vi "Test Configure.vi"(0 "niDTS BT Rx Test in":refnum<class "niDTS BT Rx Test.lvclass">, 11 "error in (no error)":errorcluster) -> (4 "niDTS BT Rx Test out":refnum<class "niDTS BT Rx Test.lvclass">, 15 "error out":errorcluster)   [LabVIEW 2015, in "niDTS BT.lvlib" / "niDTS BT Rx Test.lvclass"]
uses:
  niDTS BT Rx Test.lvclass
  Includes/niDTS BT DUT INC Parameters.ctl
  RiviInstDriver/niRfsgBT/Includes/niRfsgBt INC Handle.ctl
  RiviInstDriver/niRfsgBT/Objects/niRfsgBt.lvclass
  niDTS BT Rx Test.lvclass/niDTS BT Rx Test.ctl
  RiviInstDriver/InstDriver/Objects/InstDriver.lvclass/InstDriver.ctl
  RiviInstDriver/InstDriver/Objects/Read VISA resource.vi
  RiviInstDriver/InstDriver/Objects/Set VISA Read (Byte Count).vi
  TestStand/Station/Objects/SystemTechnologyCatalog/niDTS SystemTechnologyCatalog.lvclass
  TestStand/Station/Objects/SystemDut/niDTS SystemDut.lvclass
  Framework/Dut/Objects/BASE_class/niDTS Dut.lvclass
  Instrument/INSTR RX/niDTS BT INSTR RX.lvclass
  Framework/niDTS Framework.lvlib
  niDTS BT.lvlib
  TestStand/niDTS TestStand.lvlib
  RiviInstDriver/InstDriver/Objects/InstDriver.lvclass
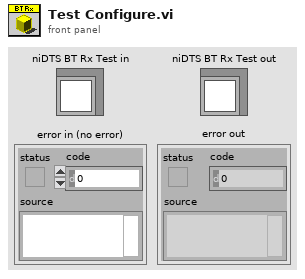
[diagram p1: front panel]
types:
  T1 = typedef "niRfsgBt.lvclass/niRfsgBT INC Handle.ctl" = refnum<data-value>
  T2 = typedef "niDTS BT.lvlib/niDTS BT DUT INC Parameters.ctl" = cluster{"Channel":i32, "Pattern":enum16{"0", "1", "01", "00001111", "PN9"}, "Packet type":enum16{"NULL", "POLL", "FHS", "DM1", "DH1", "HV1", "HV2", "HV3", "EV3", "DV", "AUX1", "DM3", "DH3", "EV4", "EV5", "DM5", "DH5", "LE-TP"}, "Power":dbl, "Report Period (ms)":dbl, "BD Address":i64, "Data Rate":enum16{"1", "2", "3"}, "Number of Packets":i32, "Packet Length, bytes":i32}
  T3 = typedef "niDTS Framework.lvlib/niDTS Dut INC Handle.ctl" = refnum<data-value>
  T4 = typedef "niDTS BT.lvlib/niDTS BT Rx Test INC Parameters.ctl" = cluster{"Channel":i32, "Dut Tx Power":dbl, "External Attenuation (dB)":dbl[], "Data Rate":enum16{"1", "2", "3"}, "Packet type":T5, "Payload Data":T6, "Carrier Mode":T7, "Number of Packets":i32, "Report Period (ms)":dbl, "BD ADDRESS":i64, "Dirty Tx":bool, "Corrupt Alternate CRC":bool, "Packet Header":T8, "Payload Header":T9, "Trigger":T10}
  T5 = typedef "niDTS BT.lvlib/niDTS BT INC Packet Type.ctl" = enum16{"NULL", "POLL", "FHS", "DM1", "DH1", "HV1", "HV2", "HV3", "EV3", "DV", "AUX1", "DM3", "DH3", "EV4", "EV5", "DM5", "DH5", "LE-TP"}
  T6 = typedef "niDTS BT.lvlib/niDTS BT Tx Test INC BD Payload Data.ctl" = enum16{"0", "1", "01", "00001111", "PN9", "AUTO"}
  T7 = typedef "niDTS BT.lvlib/niDTS BT Rx Test INC Carrier Mode.ctl" = enum16{"Burst", "Continuous"}
  T8 = typedef "niDTS BT.lvlib/niDTS BT Rx Test INC Packet Header.ctl" = cluster{"LT Address":i8, "Flow":i8, "ARQN":enum16{"NAK", "ACK"}, "Sequence Bit":i8}
  T9 = typedef "niDTS BT.lvlib/niDTS BT Rx Test INC Payload Header.ctl" = cluster{"LCh":i32, "HeaderFlowControlBit":bool, "Length (-1 AutoSet Max)":i32}
  T10 = typedef "niDTS BT.lvlib/niDTS BT DUT INC SG Trigger.ctl" = cluster{"TriggerEdge":enum16{"RISing", "FALLing"}, "TriggerSource":enum16{"IMMediate", "PFI 0", "PFI 1", "RTSI 0", "RTSI 1", "RTSI 2", "RTSI 3", "RTSI 4", "RTSI 5", "RTSI 6", "RTSI 7", "PXI STAR", "Software"}, "TriggerDelay (sec)":dbl, "TriggerTimeout (sec)":dbl}
  T11 = typedef "InstDriver.lvclass/niInstDriver INC Handle.ctl" = refnum<data-value>
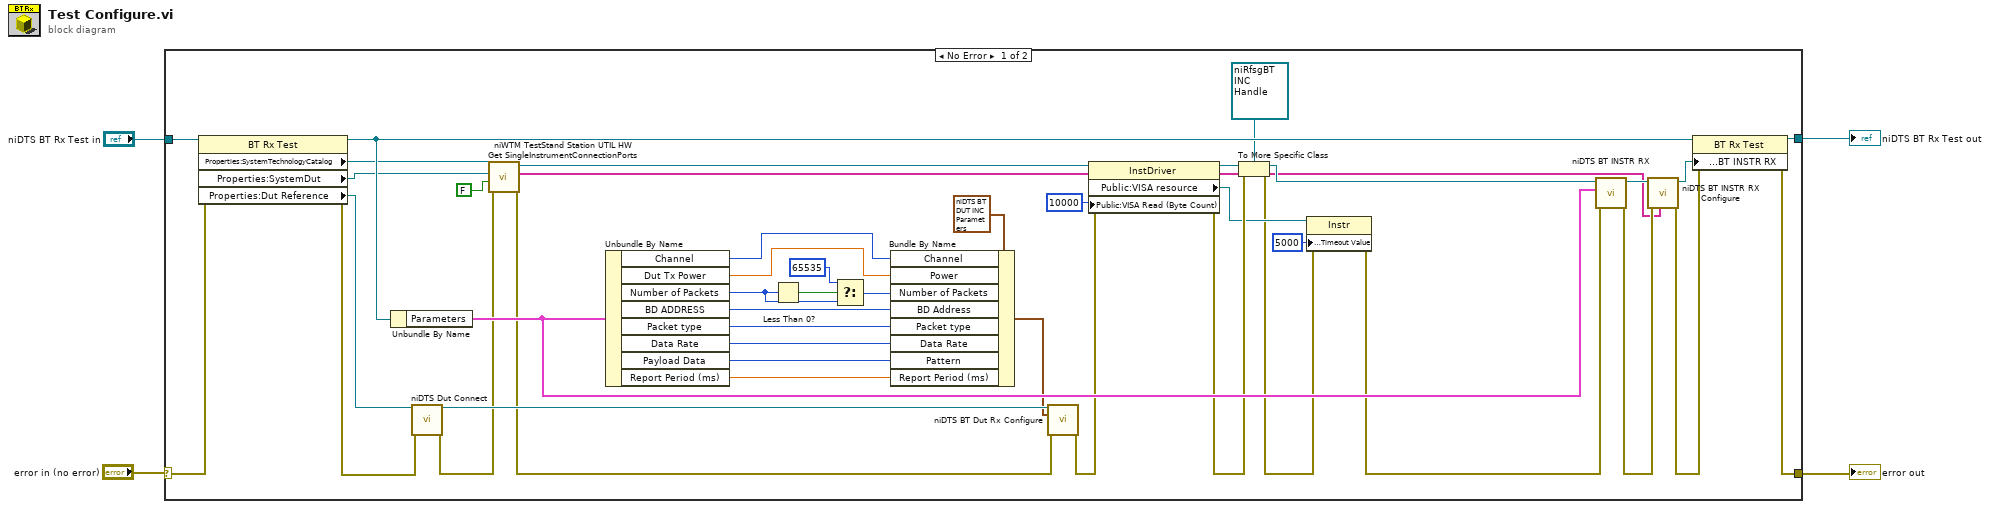
[diagram p0: block diagram]
diagram:
  n1 = case shown="No Error" "error in (no error)" {
    selector: "error in (no error)" -> [w24 w49]
    tunnel: [w32 w49] -> w3
    tunnel: [w33 w48] -> w2
    tunnel: "niDTS BT Rx Test in" -> [w47 w48]
    frame No Error {
      n2 = property class="BT Rx Test"(reference=w47, error in=w24) -> (reference out=w25:refnum<class "niDTS BT Rx Test.lvclass">, error out=w23:errorcluster, "Properties:SystemTechnologyCatalog"=w21:refnum<class "niDTS SystemTechnologyCatalog.lvclass">, "Properties:SystemDut"=w20:refnum<class "niDTS SystemDut.lvclass">, "Properties:Dut Reference"=w46:T3)
      n3 = Unbundle By Name(w25) -> ("Parameters"=w38:T4)
      n4 = call "niDTS Dut Connect.vi"("Dut Handle"=w46, "error in (no error)"=w23) -> ("Dut Handle out"=w45:T3, "error out"=w19:errorcluster)  [unwired: 12 in]
      n5 = call "niWTM TestStand Station UTIL HW Get SingleInstrumentConnectionPorts.vi"("error in (no error)"=w19, "TX Instrument"=FALSE, "SystemDut"=w20, "SystemTechnologyCatalog"=w21) -> ("error out"=w16:errorcluster, "Ports"=w5:string[], "InstDriver Handle"=w18:T11)  [unwired: 5 in]
      n6 = Unbundle By Name(w38) -> ("Channel"=w26:i32, "Dut Tx Power"=w27:dbl, "Number of Packets"=w29:i32, "BD ADDRESS"=w7:i64, "Packet type"=w43:T5, "Data Rate"=w42:enum16{"1", "2", "3"}, "Payload Data"=w41:T6, "Report Period (ms)"=w40:dbl)
      n7 = Less Than 0?(x=w29) -> (x < 0?=w30:bool)
      n8 = Select(t=65535, s=w30, f=w29) -> (s? t:f=w6:i32)
      n9 = Bundle By Name(cluster=T2 {"Channel"=36, "Pattern"=enum."01", "Packet type"=enum."DH1", "Power"=0.0, "Report Period (ms)"=1000.0, "BD Address"=1500, "Data Rate"=enum."2", "Number of Packets"=1500, "Packet Length, bytes"=-1} ("niDTS BT DUT Parameters"), "Channel"=w26, "Power"=w27, "Number of Packets"=w6, "BD Address"=w7, "Packet type"=w43, "Data Rate"=w42, "Pattern"=w41, "Report Period (ms)"=w40) -> (w22:T2)
      n10 = call "niDTS BT Dut Rx Configure.vi"("Dut Handle in"=w45, "niDTS BT DUT Parameters"=w22, "error in (no error)"=w16) -> ("error out"=w15:errorcluster)  [unwired: 11 in, 1 out]
      n11 = property class="InstDriver"(reference=w18, error in=w15, "Public:VISA Read (Byte Count)"=u32 10000 ("VISA Read (Byte Count)")) -> (reference out=w11:T11, error out=w14:errorcluster, "Public:VISA resource"=w13:refnum<visa-resource-name>)
      n12 = To More Specific Class(target class=T1 refnum ("niRfsgBT Handle"), reference=w11, error in=w14) -> (specific class reference=w9:T1, error out=w12:errorcluster)
      n13 = property class="Instr"(reference=w13, error in=w12, "General Settings:Timeout Value"=u32 5000) -> (error out=w35:errorcluster)  [unwired: 1 out]
      n14 = call "niDTS BT INSTR RX.vi"("error in (no error)"=w35, "BT Rx Input Parameters"=w38, "niRfsgBT Handle"=w9) -> ("error out"=w37:errorcluster, "niDTS BT INSTR RX out"=w36:refnum<class "niDTS BT INSTR RX.lvclass">)  [unwired: 7 in]
      n15 = call-dynamic "niDTS BT INSTR RX Configure.vi"("Ports"=w5, "error in (no error)"=w37, "niDTS BT INSTR RX in"=w36) -> ("error out"=w31:errorcluster, "niDTS BT INSTR RX out"=w34:refnum<class "niDTS BT INSTR RX.lvclass">)  [unwired: 7 in]
      n16 = property class="BT Rx Test"(reference=w25, error in=w31, "Properties:Results:BT INSTR RX"=w34) -> (reference out=w33:refnum<class "niDTS BT Rx Test.lvclass">, error out=w32:errorcluster)
    }
    frame Error {
    }
  }
  "error out" <- w3
  "niDTS BT Rx Test out" <- w2
